vi "Finish.vi"   [LabVIEW 2014]
doc: "This VI is called just before exiting. It is expected to close I/O refnum, save collected data, etc."
uses:
  Global Ref.vi
types:
  T1 = typedef "Global Ref typedef.ctl" = cluster{"Drive":cluster{"RobotDriveDevRef":T2}, "Joysticks":cluster{"JoyDriveRef":T12, "JoyOpRef":T12, "JoySabatourRef":T12}, "Lift":cluster{"LiftMotorRefLeft":T3, "LiftMotorRefRight":T3}, "Lift Limits":cluster{"Bottom Left":T14, "Bottom Right":T14}, "Accel":cluster{"AccelerometerDevRef":T16}, "Lift Encoder":cluster{"AIDeviceRefRight":T25, "AIDeviceRefLeft":T25}, "Lights":cluster{"Swag Light Ref cluster":cluster{"PWMDeviceRef1":T26, "PWMDeviceRef2":T26, "PWMDeviceRef3":T26, "PWMDeviceRef4":T26, "PWMDeviceRef5":T26, "PWMDeviceRef6":T26, "PWMDeviceRef7":T26, "PWMDeviceRef8":T26}}, "Camera":cluster{"GrayScaleImage":T27, "ColorImage":T27, "CameraDevRef":T28}, "Drive Encoders":cluster{"AIDeviceRef Left":T25, "AIDeviceRef Right":T25}, "Gyro":cluster{"GyroDevRef":T29}, "Relay":cluster{"RelayDevRef":T30, "RelayDevRef 2":T30}, "Gripper Arm Motors":cluster{"Gripper Arm Left":T3, "Gripper Arm Right":T3}}
  T2 = typedef "WPI_RobotDriveDevRef.ctl" = cluster{"DevStatus":errorcluster, "Motors[]":T3[], "Square Inputs":bool, "Max Output":dbl}
  T3 = typedef "WPI_MotorControlDeviceRef.ctl" = cluster{"DeviceStatus":errorcluster, "Type":T4, "PWM":cluster{"Controller":T5, "PWM Channel":T6, "DeadBand":T7}, "CAN":cluster{"Device Number":u8, "Control Mode":T8, "Semaphore":T9, "Max Vout":dbl, "TalonSRX Control Mode":T10}, "Invert":bool, "TransformRef":T11, "InvTransformRef":T11}
  T4 = typedef "WPI_MotorControlType.ctl" = enum16{"PWM", "CAN", "CANTalonSRX"}
  T5 = typedef "FPGA_TypedefDigitalModule.ctl" = enum16{"Controller 1"}
  T6 = typedef "FPGA_DIOPWMChannel.ctl" = enum8{"PWM 0", "PWM 1", "PWM 2", "PWM 3", "PWM 4", "PWM 5", "PWM 6", "PWM 7", "PWM 8", "PWM 9", "PWM MXP 0", "PWM MXP 1", "PWM MXP 2", "PWM MXP 3", "PWM MXP 4", "PWM MXP 5", "PWM MXP 6", "PWM MXP 7", "PWM MXP 8", "PWM MXP 9", "Invalid"}
  T7 = typedef "WPI_PWMDeadband.ctl" = cluster{"Name":string, "maxPositivePwm":i32, "minPositivePwm":i32, "centerPwm":i32, "maxNegativePwm":i32, "minNegativePwm":i32, "angularRange":u16}
  T8 = typedef "WPI_CANJaguar_ControlMode.ctl" = enum8{"Percent VBus", "Current", "Speed", "Position", "Voltage"}
  T9 = typedef "Semaphore RefNum" = refnum<k1>
  T10 = typedef "WPI_CANTalonSRX_APIControlMode.ctl" = enum8{"Percent VBus", "Speed", "Position", "Slave", "Unchanged / Invalid"}
  T11 = typedef "WPI_PWMTransform_ConPane.ctl" = refnum<vi>
  T12 = typedef "WPI_JoystickDevRef.ctl" = cluster{"Device":T13}
  T13 = typedef "WPI_JoystickDeviceEnum.ctl" = enum16{"USB 0", "USB 1", "USB 2", "USB 3", "USB 4", "USB 5"}
  T14 = typedef "WPI_DigitalInputDevRef.ctl" = cluster{"DevStatus":errorcluster, "DIO Channel":T15, "Controller":T5}
  T15 = typedef "FPGA_DIOChannel.ctl" = enum8{"DIO 0", "DIO 1", "DIO 2", "DIO 3", "DIO 4", "DIO 5", "DIO 6", "DIO 7", "DIO 8", "DIO 9", "DIO MXP 0", "DIO MXP 1", "DIO MXP 2", "DIO MXP 3", "DIO MXP 4", "DIO MXP 5", "DIO MXP 6", "DIO MXP 7", "DIO MXP 8", "DIO MXP 9", "DIO MXP 10", "DIO MXP 11", "DIO MXP 12", "DIO MXP 13", "DIO MXP 14", "DIO MXP 15", "Invalid"}
  T16 = typedef "WPI_AccelerometerDevRef.ctl" = cluster{"DevStatus":errorcluster, "Controller":T17, "Scaling":T18, "Analog Channels":T19, "I2C Bus":T21, "SPI Bus":T22, "Accel Range":T23, "ADXL345 Axes":T24, "Handle":i32, "Device Address":u8, "Accel Type":enum16{"Analog", "ADXL345 I2C", "ADXL345 SPI", "Internal"}}
  T17 = typedef "FPGA_TypedefAnalogModule.ctl" = enum16{"Controller 1"}
  T18 = typedef "WPI_AccelerometerScaling.ctl" = cluster{"Gain (VoltsPerG)":dbl, "Center Voltage":dbl}
  T19 = typedef "WPI_AccelerometerAnalogChannels.ctl" = cluster{"X-Axis":T20, "Y-Axis":T20, "Z-Axis":T20}
  T20 = typedef "FPGA_AIChannel.ctl" = enum8{"AI 0", "AI 1", "AI 2", "AI 3", "AI MXP 0", "AI MXP 1", "AI MXP 2", "AI MXP 3", "Invalid"}
  T21 = typedef "i2c_bus.ctl" = enum16{"I2C On-Board", "I2C MXP", "Invalid"}
  T22 = typedef "spi_bus.ctl" = enum16{"SPI On-Board, CS0", "SPI On-Board, CS1", "SPI On-Board, CS2", "SPI On-Board, CS3", "SPI MXP", "Invalid"}
  T23 = typedef "ADXL345 Range.ctl" = u8
  T24 = typedef "WPI_AccelerometerADXL345 Axes.ctl" = cluster{"X-Axis":bool, "Y-Axis":bool, "Z-Axis":bool}
  T25 = typedef "WPI_AnalogChannelDevRef.ctl" = cluster{"DevStatus":errorcluster, "Controller":T17, "Analog Channel":T20}
  T26 = typedef "WPI_PWMDeviceRef.ctl" = cluster{"DeviceStatus":errorcluster, "Controller":T5, "PWM Channel":T6}
  T27 = typedef "IMAQ Image.ctl" = refnum<image>
  T28 = typedef "WPI_CameraDevRef.ctl" = cluster{"Camera Address":string, "CameraStatus":errorcluster}
  T29 = typedef "WPI_GyroDevRef.ctl" = cluster{"DevStatus":errorcluster, "Analog Module":T17, "Analog Channel":T20, "Offset":dbl, "Gain (VoltsPerDegree/Second)":dbl}
  T30 = typedef "WPI_RelayDevRef.ctl" = cluster{"DevStatus":errorcluster, "Relay Channel":T31, "Controller":T5, "Relay Direction":T32}
  T31 = typedef "FPGA_DIORelayChannel.ctl" = enum8{"Relay 0", "Relay 1", "Relay 2", "Relay 3", "Invalid"}
  T32 = typedef "WPI_RelayDirection.ctl" = enum16{"Both directions", "Forward only", "Reverse only"}
  T33 = cluster{"PWMDeviceRef1":T26, "PWMDeviceRef2":T26, "PWMDeviceRef3":T26, "PWMDeviceRef4":T26, "PWMDeviceRef5":T26, "PWMDeviceRef6":T26, "PWMDeviceRef7":T26, "PWMDeviceRef8":T26}
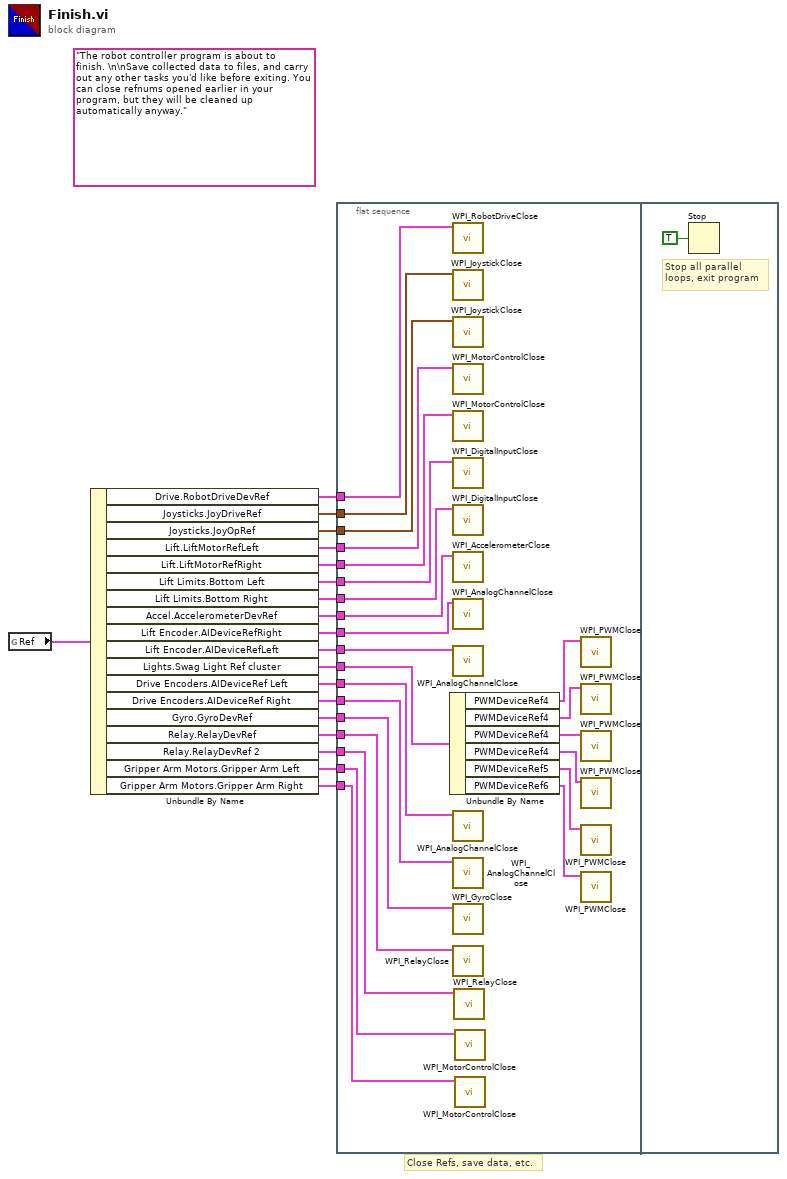
[diagram p0: block diagram]
diagram:
  (unwired) "The robot controller program is about to finish. \n\nSave collected data to files, and carry out any other tasks you'd like before exiting. You can close refnums opened earlier in your program, but they will be cleaned up automatically anyway."
  # "Close Refs, save data, etc."
  n1 = global read "Global Ref.vi" "Ref"() -> (w19:T1)
  n2 = Unbundle By Name(w19) -> ("Drive.RobotDriveDevRef"=w18:T2, "Joysticks.JoyDriveRef"=w17:T12, "Joysticks.JoyOpRef"=w16:T12, "Lift.LiftMotorRefLeft"=w15:T3, "Lift.LiftMotorRefRight"=w14:T3, "Lift Limits.Bottom Left"=w13:T14, "Lift Limits.Bottom Right"=w12:T14, "Accel.AccelerometerDevRef"=w11:T16, "Lift Encoder.AIDeviceRefRight"=w10:T25, "Lift Encoder.AIDeviceRefLeft"=w9:T25, "Lights.Swag Light Ref cluster"=w8:T33, "Drive Encoders.AIDeviceRef Left"=w7:T25, "Drive Encoders.AIDeviceRef Right"=w6:T25, "Gyro.GyroDevRef"=w5:T29, "Relay.RelayDevRef"=w4:T30, "Relay.RelayDevRef 2"=w3:T30, "Gripper Arm Motors.Gripper Arm Left"=w2:T3, "Gripper Arm Motors.Gripper Arm Right"=w1:T3)
  n3 = flat-sequence {
    tunnel: w18 -> [w43]
    tunnel: w17 -> [w42]
    tunnel: w16 -> [w41]
    tunnel: w15 -> [w40]
    tunnel: w14 -> [w39]
    tunnel: w13 -> [w38]
    tunnel: w12 -> [w37]
    tunnel: w11 -> [w36]
    tunnel: w10 -> [w35]
    tunnel: w9 -> [w34]
    tunnel: w8 -> [w33]
    tunnel: w7 -> [w26]
    tunnel: w6 -> [w25]
    tunnel: w5 -> [w24]
    tunnel: w4 -> [w23]
    tunnel: w3 -> [w22]
    tunnel: w2 -> [w20]
    tunnel: w1 -> [w21]
    frame #0 {
      n4 = Unbundle By Name(w33) -> ("PWMDeviceRef4"=w32:T26, "PWMDeviceRef4"=w31:T26, "PWMDeviceRef4"=w30:T26, "PWMDeviceRef4"=w29:T26, "PWMDeviceRef5"=w28:T26, "PWMDeviceRef6"=w27:T26)
      n5 = call <vilib>:"WPI_RobotDriveClose.vi"("RobotDriveDevRef"=w43) -> ()  [unwired: 10 in, 1 out]
      n6 = call <vilib>:"WPI_JoystickClose.vi"("JoystickDevRef"=w42) -> ()  [unwired: 11 in]
      n7 = call <vilib>:"WPI_JoystickClose.vi"("JoystickDevRef"=w41) -> ()  [unwired: 11 in]
      n8 = call <vilib>:"WPI_MotorControlClose.vi"("MotorControlDevRef"=w40) -> ()  [unwired: 10 in, 1 out]
      n9 = call <vilib>:"WPI_MotorControlClose.vi"("MotorControlDevRef"=w39) -> ()  [unwired: 10 in, 1 out]
      n10 = call <vilib>:"WPI_DigitalInputClose.vi"("DigitalInputDevRef"=w38) -> ()  [unwired: 10 in, 1 out]
      n11 = call <vilib>:"WPI_DigitalInputClose.vi"("DigitalInputDevRef"=w37) -> ()  [unwired: 10 in, 1 out]
      n12 = call <vilib>:"WPI_AccelerometerClose.vi"("AccelerometerDevRef"=w36) -> ()  [unwired: 10 in, 1 out]
      n13 = call <vilib>:"WPI_AnalogChannelClose.vi"("AIDeviceRef"=w35) -> ()  [unwired: 10 in, 1 out]
      n14 = call <vilib>:"WPI_AnalogChannelClose.vi"("AIDeviceRef"=w34) -> ()  [unwired: 10 in, 1 out]
      n15 = call <vilib>:"WPI_AnalogChannelClose.vi"("AIDeviceRef"=w26) -> ()  [unwired: 10 in, 1 out]
      n16 = call <vilib>:"WPI_AnalogChannelClose.vi"("AIDeviceRef"=w25) -> ()  [unwired: 10 in, 1 out]
      n17 = call <vilib>:"WPI_GyroClose.vi"("GyroDevRef"=w24) -> ()  [unwired: 10 in, 1 out]
      n18 = call <vilib>:"WPI_RelayClose.vi"("RelayDevRef"=w23) -> ()  [unwired: 10 in, 1 out]
      n19 = call <vilib>:"WPI_RelayClose.vi"("RelayDevRef"=w22) -> ()  [unwired: 10 in, 1 out]
      n20 = call <vilib>:"WPI_MotorControlClose.vi"("MotorControlDevRef"=w20) -> ()  [unwired: 10 in, 1 out]
      n21 = call <vilib>:"WPI_MotorControlClose.vi"("MotorControlDevRef"=w21) -> ()  [unwired: 10 in, 1 out]
      n22 = call <vilib>:"WPI_PWMClose.vi"("PWMDeviceRef"=w32) -> ()  [unwired: 10 in, 1 out]
      n23 = call <vilib>:"WPI_PWMClose.vi"("PWMDeviceRef"=w31) -> ()  [unwired: 10 in, 1 out]
      n24 = call <vilib>:"WPI_PWMClose.vi"("PWMDeviceRef"=w30) -> ()  [unwired: 10 in, 1 out]
      n25 = call <vilib>:"WPI_PWMClose.vi"("PWMDeviceRef"=w29) -> ()  [unwired: 10 in, 1 out]
      n26 = call <vilib>:"WPI_PWMClose.vi"("PWMDeviceRef"=w28) -> ()  [unwired: 10 in, 1 out]
      n27 = call <vilib>:"WPI_PWMClose.vi"("PWMDeviceRef"=w27) -> ()  [unwired: 10 in, 1 out]
    }
    frame #1 {
      # "Stop all parallel\nloops, exit program"
      n28 = Stop(stop? (T)=TRUE ("Quit")) -> ()
    }
  }
